vi "Update Item.vi"(8 "error in (no error)":errorcluster, 9 "New Item":refnum<class "Data Item.lvclass">, 10 "Tag":string, 11 "Tree Manager in":refnum<class "Tree Manager.lvclass">) -> (0 "error out":errorcluster, 3 "Tree Manager out":refnum<class "Tree Manager.lvclass">)   [LabVIEW 2018, in "VILab.lvlib" / "Tree Manager.lvclass"]
uses:
  Tree Manager.lvclass
  Data Item.lvclass
panel:
  in  "Update children? (T)":bool=TRUE
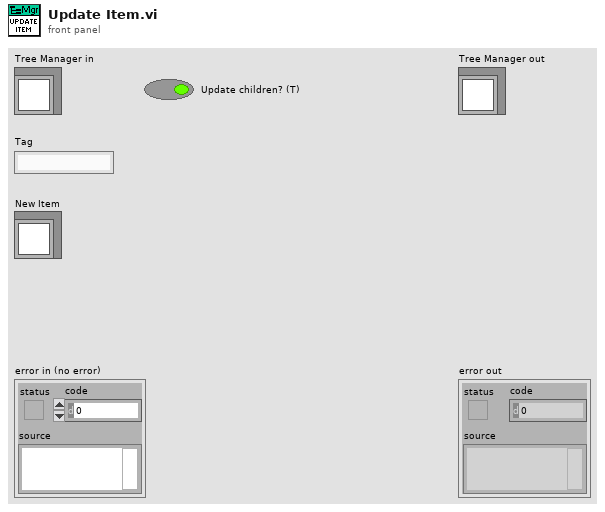
[diagram p1: front panel]
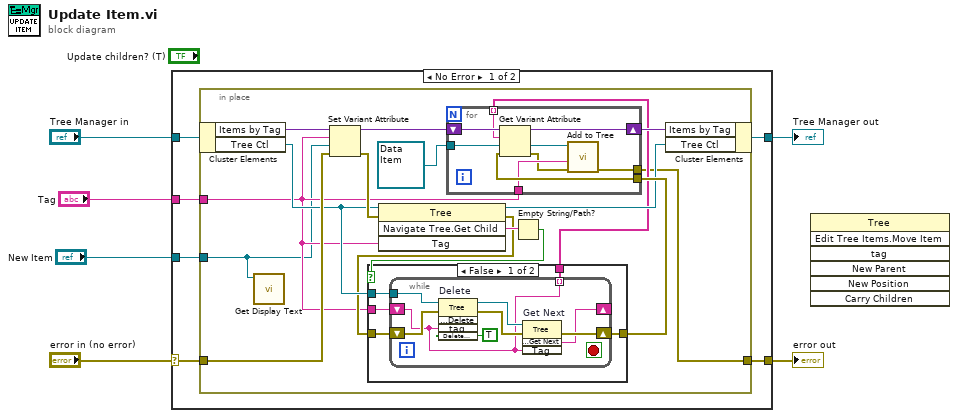
[diagram p0: block diagram]
diagram:
  n1 = case shown="No Error" "error in (no error)" {
    selector: "error in (no error)" -> [w9 w53]
    tunnel: [w7 w53] -> w5
    tunnel: [w10 w52] -> w3
    tunnel: "Tree Manager in" -> [w12 w52]
    tunnel: "Tag" -> [w11 _]
    tunnel: "New Item" -> [w8 _]
    frame No Error {
      n2 = in-place {
        in-place-border: w11 -> [w20]
        in-place-border: w9 -> [w27]
        in-place-border: w8 -> [w13]
        in-place-border: [w14] -> w7
        n3 = in-place-cluster #1(w12) -> ("Items by Tag"=w28:variant, "Tree Ctl"=w23:refnum<vi>)
        n4 = call-dynamic "Get Display Text.vi"("Data Item in"=w13) -> ()  [unwired: 7 in, 4 out]
        n5 = Set Variant Attribute(Variant=w28, name=w20, value=w13, error in=w27) -> (Variant out=w21:variant, error out=w26:errorcluster)  [unwired: 1 out]
        n6 = invoke class="Tree" method="Navigate Tree.Get Child"(reference=w23, error in=w26, "Tag"=w20) -> (reference out=w17:refnum<vi>, error out=w22:errorcluster, "Navigate Tree:Get Child"=w25:string)  [unwired: 1 in, 1 out]
        n7 = Empty String/Path?(string/path=w25) -> (empty?=w24:bool)
        n8 = case shown="False" w24 {
          tunnel: w20 -> [w42 _]
          tunnel: w23 -> [w41 _]
          tunnel: w22 -> [w40 w51]
          tunnel: [w39 w51] -> w19
          tunnel: [w38 _] -> w15
          frame False {
            n9 = while {
              shift-right: [w44] -> _
              shift-left: w42 -> [w43]
              tunnel: w41 -> [w50]
              shift-right: [w45] -> w39
              shift-left: w40 -> [w46]
              tunnel: [w43] -> w38 mode=indexing
              stop <- _ stop-if-true
              n10 = invoke on="Delete" class="Tree" method="Edit Tree Items.Delete"(reference=w50, error in=w46, "tag"=w43, "Delete Children"=TRUE ("Delete Children?")) -> (reference out=w48:refnum<vi>, error out=w47:errorcluster)  [unwired: 1 in, 3 out]
              n11 = invoke on="Get Next" class="Tree" method="Navigate Tree.Get Next"(reference=w48, error in=w47, "Tag"=w43) -> (error out=w45:errorcluster, "Navigate Tree:Get Next Item"=w44:string)  [unwired: 1 in, 2 out]
            }
          }
          frame True {
          }
        }
        n12 = for {
          tunnel: w20 -> [w32]
          tunnel: w19 -> [w36]
          shift-right: [w35] -> w18
          shift-left: w21 -> [w37]
          tunnel: refnum<class "Data Item.lvclass"> refnum ("VILab.lvlib:Data Item.lvclass") -> [w34]
          tunnel: w15 -> [w31] mode=indexing
          tunnel: [w29] -> w14
          n13 = Get Variant Attribute(Variant=w37, name=w31, default value (empty Variant)=w34, error in=w36) -> (duplicate Variant=w35:variant, value=w33:refnum<class "Data Item.lvclass">, error out=w30:errorcluster)  [unwired: 1 out]
          n14 = call-dynamic "Add to Tree.vi"("error in (no error)"=w30, "Parent Tag"=w32, "Data Item in"=w33) -> ("error out"=w29:errorcluster)  [unwired: 6 in, 2 out]
        }
        n15 = in-place-cluster #1("Items by Tag"=w18, "Tree Ctl"=w17) -> (w10:refnum<class "Tree Manager.lvclass">)
      }
    }
    frame Error {
    }
  }
  "error out" <- w5
  "Tree Manager out" <- w3
  n16 = invoke class="Tree" method="Edit Tree Items.Move Item"() -> ()  [unwired: 7 in, 7 out]
